vi "ADC_GetDataVoltCh.vi"(8 "error in (no error)":errorcluster, 10 "Data":dbl, 11 "wCh":i16) -> (0 "error out":errorcluster, 2 "Data out":dbl, 3 "function return":i16)   [LabVIEW 2013, in "HS3AcquireData.lvlib"]
doc: "Description: This routine transfers the measured data of one channel from the acquisition memory in the hardware via the DLL into the memory in the application. The measured data is returned in volt. dData is an array. The caller must ensure that there is enough space in the array to contain the data. Therefore the size of the array in bytes must be at least RecordLength * sizeof( double )\nInput: wCh Indicates from which channel the data has to be\nretrieved\nOutput: dData The array to which the measured data of the\nrequested channel should be passed.\nReturn value E_NO_ERRORS | E_NO_HARDWARE\n\nFunction prototype: word ADC_GetDataVoltCh( word wCh, double *Data )\n\nshort int ADC_GetDataVoltCh ( short int wCh, double *Data );"
uses:
  HS3AcquireData.lvlib
  hs3.dll
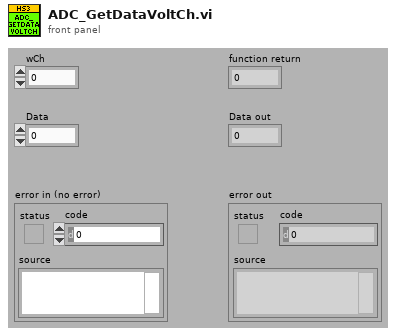
[diagram p1: front panel]
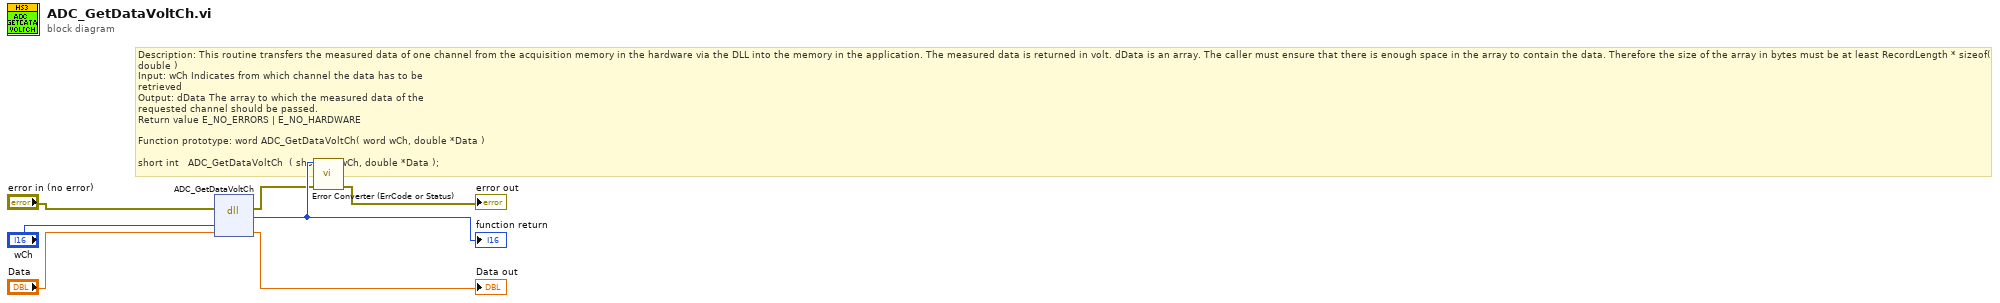
[diagram p0: block diagram]
diagram:
  # "Description: This routine transfers the measured data of one channel from the acquisition memory in the hardware via the DLL into the memory in the application. The measured data is returned in volt. dData is an array. The caller must ensure that there is enough space in the array to contain the data. Therefore the size of the array in bytes must be at least RecordLength * sizeof( double )\nInput: wCh Indicates from which channel the data has to be\nretrieved\nOutput: dData The array to which the measured data of the\nrequested channel should be passed.\nReturn value E_NO_ERRORS | E_NO_HARDWARE\n\nFunction prototype: word ADC_GetDataVoltCh( word wCh, double *Data )\n\nshort int \t\tADC_GetDataVoltCh\t\t( short int wCh, double *Data );"
  n1 = dll-call lib="C:/Documents and Settings/admin/Pulpit/HS3 LabViewLib/HS3_WRAPPER/AcquireData/hs3.*" fn="ADC_GetDataVoltCh"(error in="error in (no error)", "wCh"="wCh", "Data"="Data") -> (error out=w2:errorcluster, w7:i16, "Data"=→"Data out":dbl)  [unwired: 3 in, 1 out]
  "function return" <- w7
  n2 = call "Error Converter (ErrCode or Status).vi"("error in (no error)"=w2, "error code"=w7) -> ("error out"=→"error out":errorcluster)  [unwired: 9 in]
